vi "spectrometer-wavelength-legacy.vi"(2 "set pixel width":sgl, 3 "Set Number Pixels":i32) -> (1 "wavelength array":sgl[](array[numeric]), 5 "GetCalibration":u32, 6 "Set Pixel Width":u32, 7 "Set Number Pixels":u32, 9 "Wavelength Last Pixel":sgl, 10 "Wavelength First Pixel":sgl)   [LabVIEW 2015]
uses:
  ShamrockCIF.dll
panel:
  in  "Case Constant\n(See Context Help) 3":bool=TRUE
  in  "Case Constant\n(See Context Help) 2":bool=TRUE
  in  "Case Constant\n(See Context Help)":bool=TRUE
  # "CALIBRATION"
  # "ACTIONS"
  # "SDK RETURN VALUES"
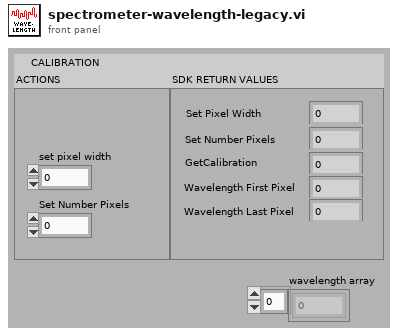
[diagram p1: front panel]
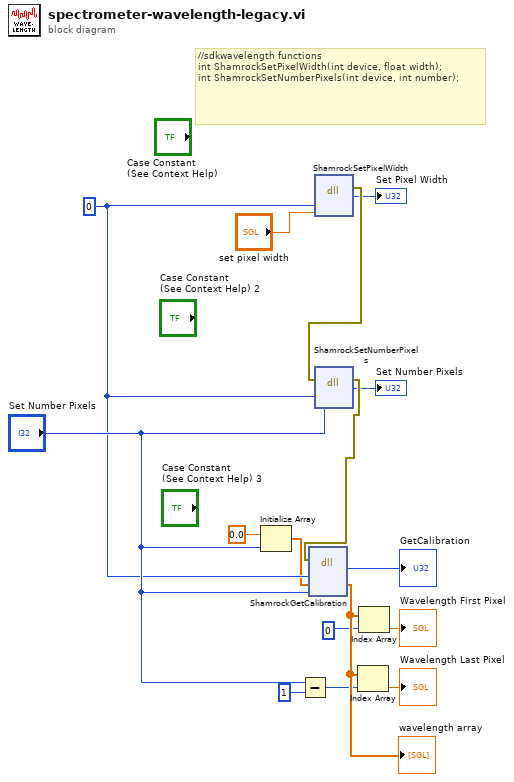
[diagram p0: block diagram]
diagram:
  w15 = 0 ("Device No")
  # "//sdkwavelength functions\nint ShamrockSetPixelWidth(int device, float width);\nint ShamrockSetNumberPixels(int device, int number);"
  n1 = Initialize Array(sgl 0.0, "Set Number Pixels") -> (w7:sgl[])
  n2 = Subtract(x="Set Number Pixels", y=1) -> (x-y=w1:i32)
  n3 = dll-call lib="ShamrockCIF.dll" fn="ShamrockSetPixelWidth"(w15, "set pixel width") -> (error out=w14:errorcluster, →"Set Pixel Width":i32)  [unwired: 5 in, 1 out]
  n4 = dll-call lib="ShamrockCIF.dll" fn="ShamrockSetNumberPixels"(error in=w14, w15, "Set Number Pixels") -> (error out=w13:errorcluster, →"Set Number Pixels":i32)  [unwired: 4 in, 1 out]
  n5 = dll-call lib="ShamrockCIF.dll" fn="ShamrockGetCalibration"(error in=w13, w15, w7, "Set Number Pixels") -> (→"GetCalibration":i32, w6:sgl[])  [unwired: 4 in, 2 out]
  "wavelength array" <- w6
  n6 = Index Array(array=w6, index=w1) -> (element=→"Wavelength Last Pixel":sgl)
  n7 = Index Array(array=w6, index=0) -> (element=→"Wavelength First Pixel":sgl)
